vi "Acquire Voltage.vi"() -> ()   [LabVIEW 2013]
panel:
  out "Waveform Chart":cluster{"Scalar":dbl, dbl}(graph)
  in  "stop":bool
  in  "Delay, s":dbl(knob)=0.1 min=0.1 max=2.0 step=0.05 scale=0.0..2.0 scale format="%#.2f"
  # "Acquire Voltage"
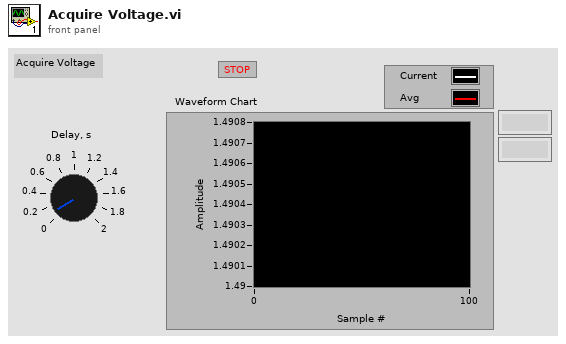
[diagram p1: front panel]
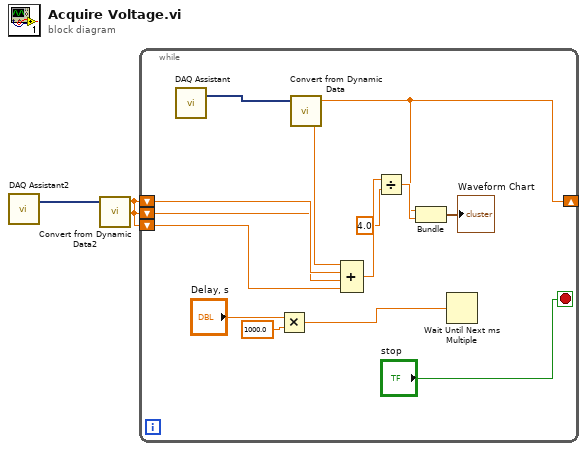
[diagram p0: block diagram]
diagram:
  n1 = call "DAQ Assistant2"() -> ("data"=w2:dynamicdata)  [unwired: 17 in, 2 out]
  n2 = call "Convert from Dynamic Data2"("Dynamic Data Type"=w2) -> ("Scalar"=w1:dbl)  [unwired: 3 in]
  n3 = while {
    shift-right: [w4] -> _
    shift-left: w1 -> [w10]
    shift-left: w1 -> [w9]
    shift-left: w1 -> [w8]
    stop <- "stop" stop-if-true
    n4 = call "DAQ Assistant"() -> ("data"=w15:dynamicdata)  [unwired: 17 in, 2 out]
    n5 = Multiply(x="Delay, s", y=1000.0) -> (x*y=w11:dbl)
    n6 = call "Convert from Dynamic Data"("Dynamic Data Type"=w15) -> ("Scalar"=w4:dbl)  [unwired: 3 in]
    n7 = Compound Arithmetic op=ADD(w4, w10, w9, w8) -> (w7:dbl)
    n8 = Divide(x=w7, y=4.0) -> (x/y=w5:dbl)
    n9 = Bundle("Scalar"=w4, w5) -> (→"Waveform Chart":cluster{"Scalar":dbl, dbl})  [unwired: 1 in]
    n10 = Wait Until Next ms Multiple(millisecond multiple=w11) -> ()  [unwired: 1 out]
  }
